vi "Errors.vi"() -> (0 "Errors":T1={"Invalid averages on scope"={"status"=FALSE, "code"=5200, "source"="Averages on scope cannot be zero. A default of 1 was used."}, "Invalid average number of points"={"status"=TRUE, "code"=5201, "source"="Average number of points cannot be zero"}, "Invalid scope readouts"={"status"=TRUE, "code"=5202, "source"="Scope readouts cannot be zero (otherwise no data would be gathered!). Default of 1 was used.\n<b> Set scope parameters</b>"}}, 1 "code array":i32[](array[numeric])=[5200, 5201, 5202], 2 "description array":string[](array[string])=["Averages on scope cannot be zero. A default of 1 was used.", "Average number of points cannot be zero", "Scope readouts cannot be zero (otherwise no data would be gathered!). Default of 1 was used.\n<b> Set scope parameters</b>"], 3 "status array":bool[](array[boolean])=[FALSE, TRUE, TRUE], 4 "call chain":string[](array[string])=["Scope.lvlib:Errors.vi"])   [LabVIEW 2017]
panel:
  in  "Define custom errors here":T1={"Invalid averages on scope"={"status"=FALSE, "code"=5200, "source"="Averages on scope cannot be zero. A default of 1 was used."}, "Invalid average number of points"={"status"=TRUE, "code"=5201, "source"="Average number of points cannot be zero"}, "Invalid scope readouts"={"status"=TRUE, "code"=5202, "source"="Set scope parameters\nScope readouts cannot be zero (otherwise no data would be gathered!). Default of 1 was used.\n<b> Set scope parameters</b>"}}
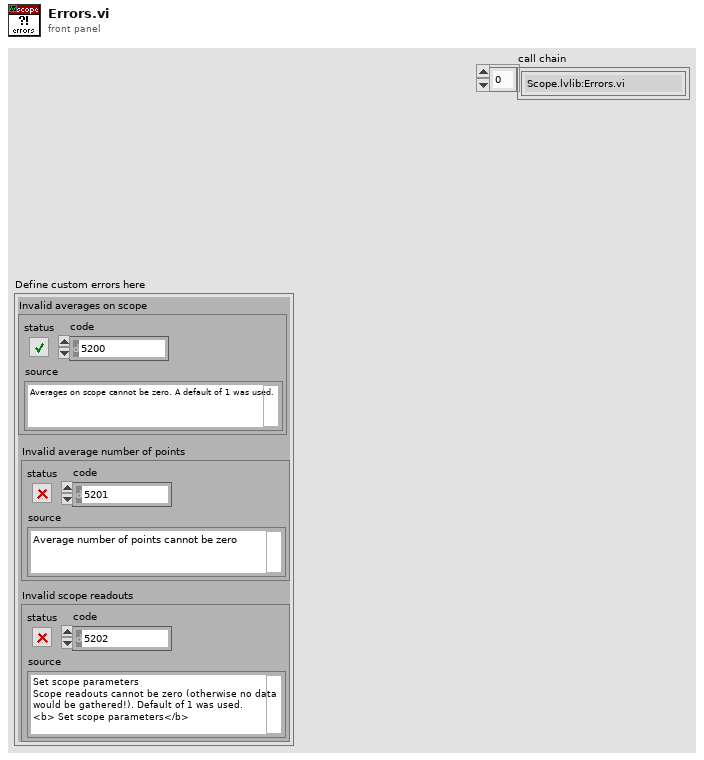
[diagram p1: front panel]
types:
  T1 = cluster{"Invalid averages on scope":errorcluster, "Invalid average number of points":errorcluster, "Invalid scope readouts":errorcluster}
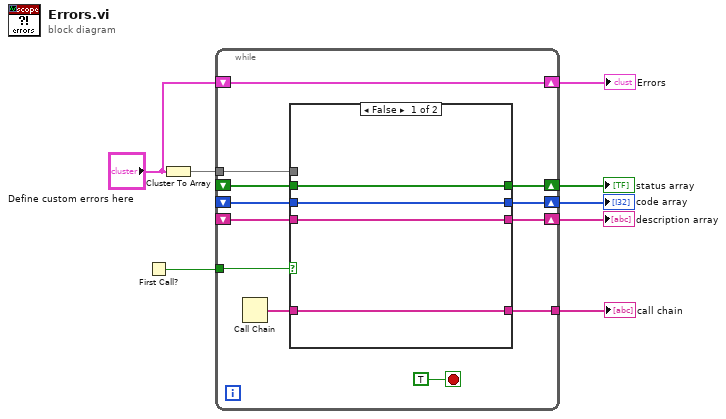
[diagram p0: block diagram]
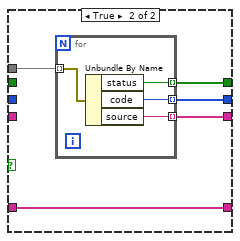
[diagram p2: hidden frame]
diagram:
  n1 = First Call?() -> (First Call?: T/F=w5:bool)
  n2 = Cluster To Array(cluster="Define custom errors here") -> (array=w4:errorcluster[])
  n3 = while {
    tunnel: w4 -> [w12]
    shift-right: [w20] -> w6
    shift-left: _ -> [w15]
    shift-right: [w19] -> w8
    shift-left: _ -> [w14]
    shift-right: [w18] -> w7
    shift-left: _ -> [w13]
    tunnel: w5 -> [w16]
    shift-right: [w11] -> w3
    shift-left: "Define custom errors here" -> [w11]
    tunnel: [w9] -> w1
    stop <- TRUE stop-if-true
    n4 = Call Chain() -> (call chain=w10:string[])
    n5 = case shown="False" w16 {
      tunnel: w12 -> [_ w29]
      tunnel: [w24 w28] -> w20
      tunnel: [w23 w27] -> w19
      tunnel: [w22 w26] -> w18
      tunnel: w15 -> [w24 _]
      tunnel: w14 -> [w23 _]
      tunnel: w13 -> [w22 _]
      tunnel: w10 -> [w21 w25]
      tunnel: [w21 w25] -> w9
      frame False {
      }
      frame True {
        n6 = for {
          tunnel: w29 -> [w33] mode=indexing
          tunnel: [w32] -> w27 mode=indexing
          tunnel: [w31] -> w26 mode=indexing
          tunnel: [w30] -> w28 mode=indexing
          n7 = Unbundle By Name(w33) -> ("status"=w30:bool, "code"=w32:i32, "source"=w31:string)
        }
      }
    }
  }
  "status array" <- w6
  "code array" <- w8
  "description array" <- w7
  "Errors" <- w3
  "call chain" <- w1
